vi "set_tilt_stage_simpler (SubVI).vi"(11 "Tot Stage Arr":dbl[](array[numeric])) -> (3 "Axes position":i32[](array[numeric]))   [LabVIEW 2016]
panel:
  out "thetaY error out":errorcluster
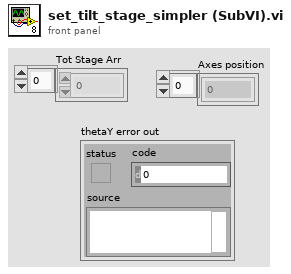
[diagram p1: front panel]
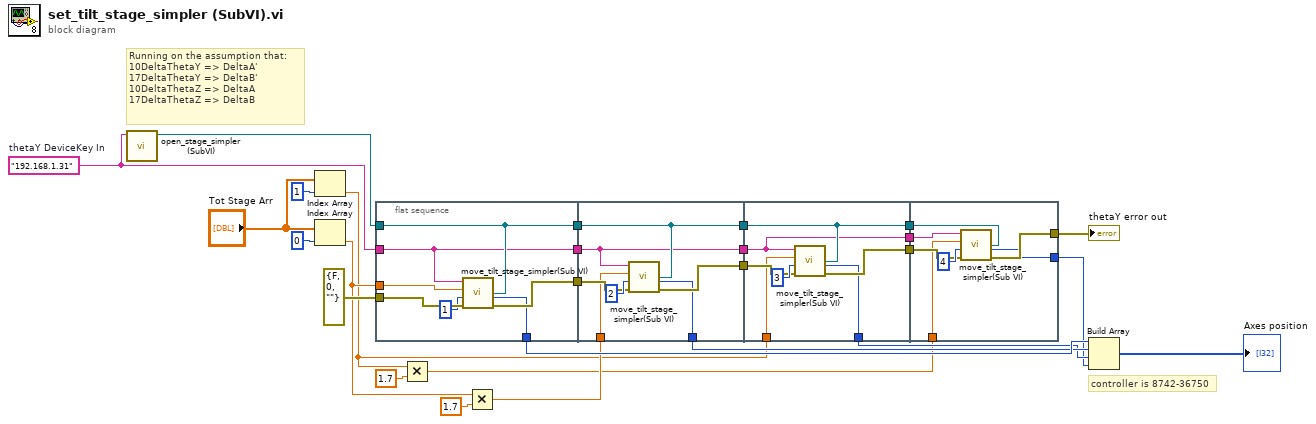
[diagram p0: block diagram]
diagram:
  w24 = "192.168.1.31"  # thetaY DeviceKey In
  # "Running on the assumption that:\n10DeltaThetaY => DeltaA'\n17DeltaThetaY => DeltaB'\n10DeltaThetaZ => DeltaA\n17DeltaThetaZ => DeltaB"
  # "controller is 8742-36750"
  n1 = call "open_stage_simpler (SubVI).vi"("IP address"=w24) -> ("reference"=w23:refnum<k24>)  [unwired: 8 in, 2 out]
  n2 = Index Array(array="Tot Stage Arr", index=1 ("index (row)")) -> (element=w2:dbl)
  n3 = Index Array(array="Tot Stage Arr", index=0 ("index (row)")) -> (element=w20:dbl)
  n4 = flat-sequence {
    tunnel: w24 -> [w30]
    tunnel: w23 -> [w31]
    tunnel: errorcluster {"status"=FALSE, "code"=0, "source"=""} ("error in (no error)") -> [w34]
    tunnel: w20 -> [w32]
    tunnel: [w31] -> w19
    tunnel: [w30] -> w16
    tunnel: [w29] -> w13
    tunnel: [w28] -> w9
    tunnel: w19 -> [w40]
    tunnel: [w40] -> w18
    tunnel: w16 -> [w39]
    tunnel: [w39] -> w15
    tunnel: w13 -> [w38]
    tunnel: [w37] -> w12
    tunnel: [w36] -> w8
    tunnel: w4 -> [w35]
    tunnel: w18 -> [w47]
    tunnel: [w47] -> w17
    tunnel: w15 -> [w46]
    tunnel: [w46] -> w14
    tunnel: w12 -> [w45]
    tunnel: [w44] -> w11
    tunnel: [w43] -> w7
    tunnel: w2 -> [w42]
    tunnel: w17 -> [w54]
    tunnel: w14 -> [w53]
    tunnel: w11 -> [w52]
    tunnel: [w51] -> w10
    tunnel: [w50] -> w6
    tunnel: w1 -> [w49]
    frame #0 {
      n5 = call "move_tilt_stage_simpler(Sub VI).vi"(".NET Refnum in"=w31, "error in (no error)"=w34, "motor"=1, "relativeSteps"=w32, "deviceKey"=w30) -> ("error out"=w29:errorcluster, "End position"=w28:i32)  [unwired: 2 out]
    }
    frame #1 {
      n6 = call "move_tilt_stage_simpler(Sub VI).vi"(".NET Refnum in"=w40, "error in (no error)"=w38, "motor"=2, "relativeSteps"=w35, "deviceKey"=w39) -> ("error out"=w37:errorcluster, "End position"=w36:i32)  [unwired: 2 out]
    }
    frame #2 {
      n7 = call "move_tilt_stage_simpler(Sub VI).vi"(".NET Refnum in"=w47, "error in (no error)"=w45, "motor"=3, "relativeSteps"=w42, "deviceKey"=w46) -> ("error out"=w44:errorcluster, "End position"=w43:i32)  [unwired: 2 out]
    }
    frame #3 {
      n8 = call "move_tilt_stage_simpler(Sub VI).vi"(".NET Refnum in"=w54, "error in (no error)"=w52, "motor"=4, "relativeSteps"=w49, "deviceKey"=w53) -> ("error out"=w51:errorcluster, "End position"=w50:i32)  [unwired: 2 out]
    }
  }
  n9 = Multiply(x=w2, y=1.7) -> (x*y=w1:dbl)
  n10 = Multiply(x=w20, y=1.7) -> (x*y=w4:dbl)
  n11 = Build Array(w9, w8, w7, w6) -> (→"Axes position":i32[])
  "thetaY error out" <- w10
